vi "Put file.vi"(8 "error in (no error)":errorcluster, 9 "Local path":path, 10 "Remote path":string, 11 "File Transfer Behavior in":refnum<class "File Transfer Behavior.lvclass">) -> (0 "error out":errorcluster, 3 "File Transfer Behavior out":refnum<class "File Transfer Behavior.lvclass">)   [LabVIEW 2015, in "RT Management.lvlib" / "File Transfer Behavior.lvclass"]
doc: "Puts the file located at \"Local path\" at \"Remote path\". The VI also creates all needed directories if the \"Remote path\" contains directories that don't exist on the target.\n\nThe recommended file path format for \"Remote path\" is \"/directory1/directory2/file.extension\". However, the VI will accept other formats and transform the path appropriately in most cases. Use the \"Strip path.vi\" and \"Build path.vi\" VIs to help with handling remote path strings."
uses:
  File Transfer Behavior.lvclass
  RT Management.lvlib
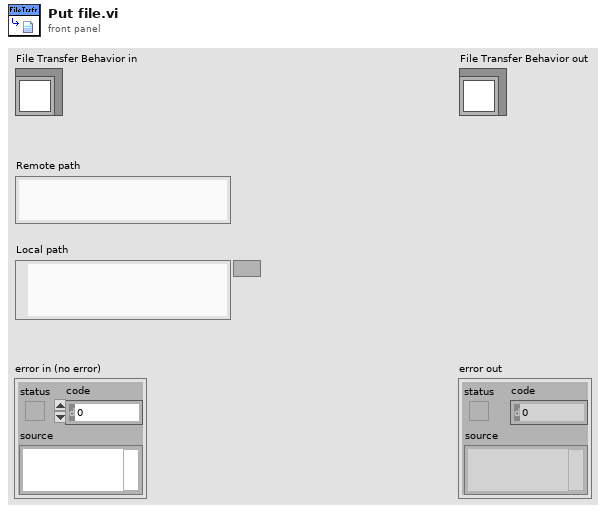
[diagram p1: front panel]
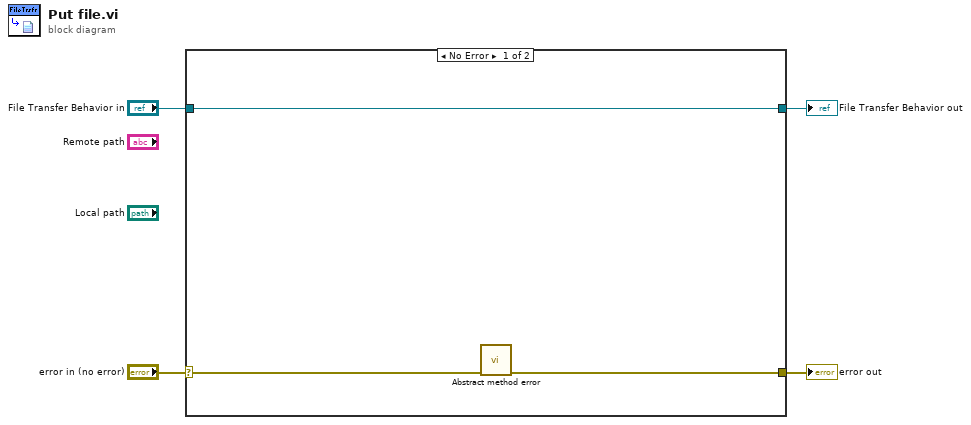
[diagram p0: block diagram]
diagram:
  n1 = case shown="No Error" "error in (no error)" {
    selector: "error in (no error)" -> [w5 w9]
    tunnel: [w6 w9] -> w3
    tunnel: [w7 w8] -> w1
    tunnel: "File Transfer Behavior in" -> [w7 w8]
    frame No Error {
      n2 = call "Abstract method error.vi"("error in (no error)"=w5) -> ("error out"=w6:errorcluster)  [unwired: 10 in]
    }
    frame Error {
    }
  }
  "error out" <- w3
  "File Transfer Behavior out" <- w1
